vi "Example Write File - Allocate String.vi"(8 "buffer":string, 9 "session id":i32, 10 "error in":errorcluster, 11 "reference in":refnum<k24>) -> (1 "string id":i32, 2 "error out":errorcluster, 3 "reference out":refnum<k24>)   [LabVIEW 2010]
uses:
  C:/tf/play/labview/Tinkerforge.dll
  Tinkerforge.dll
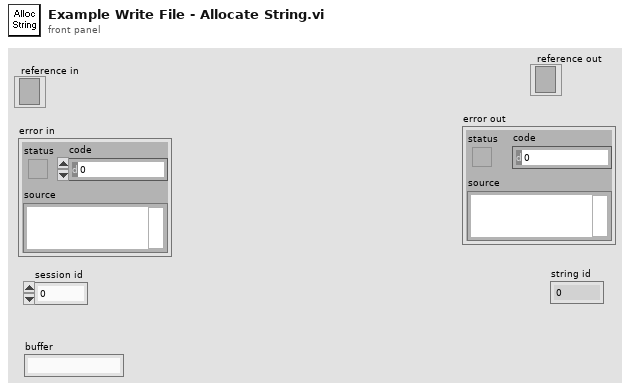
[diagram p1: front panel]
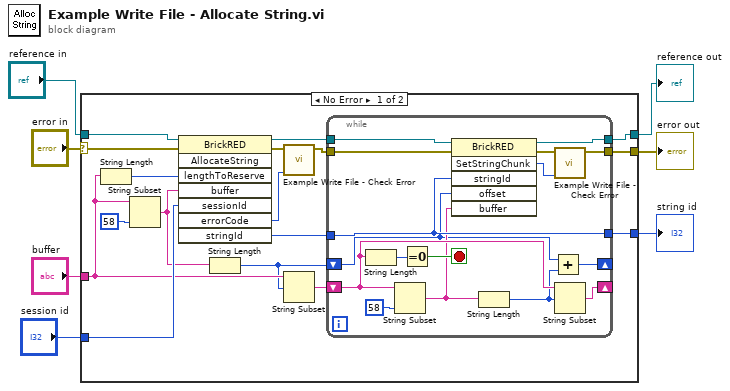
[diagram p0: block diagram]
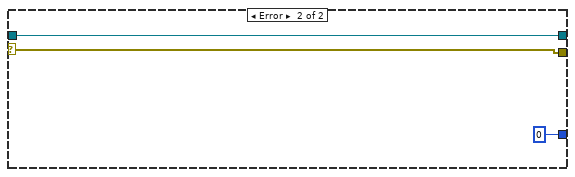
[diagram p2: hidden frame]
diagram:
  n1 = case shown="No Error" "error in" {
    selector: "error in" -> [w24 w43]
    tunnel: [w18 w43] -> w6
    tunnel: [w19 w42] -> w5
    tunnel: "reference in" -> [w23 w42]
    tunnel: "session id" -> [w22 _]
    tunnel: "buffer" -> [w15 _]
    tunnel: [w16 0 ("stringId")] -> w1
    frame No Error {
      n2 = String Length(string=w15) -> (length=w21:i32)
      n3 = String Subset(string=w15, length (rest)=58 ("length (rest)")) -> (substring=w12:string)  [unwired: 1 in]
      n4 = invoke class="BrickRED" method="AllocateString"(reference=w23, error in=w24, "lengthToReserve"=w21, "buffer"=w12, "sessionId"=w22) -> (reference out=w20:refnum<k24>, error out=w10:errorcluster, "errorCode"=w8:u8, "stringId"=w17:i32)  [unwired: 3 in, 4 out]
      n5 = String Length(string=w12) -> (length=w11:i32)
      n6 = call "Example Write File - Check Error.vi"("error code"=w8, "error in"=w10) -> ("error out"=w9:errorcluster)  [unwired: 9 in]
      n7 = String Subset(string=w15, offset (0)=w11) -> (substring=w13:string)  [unwired: 1 in]
      n8 = while {
        tunnel: w9 -> [w40]
        tunnel: [w26] -> w18
        tunnel: w20 -> [w39]
        tunnel: [w38] -> w19
        tunnel: w17 -> [w37]
        tunnel: [w37] -> w16
        shift-right: [w33] -> _
        shift-left: w13 -> [w32]
        shift-right: [w28] -> _
        shift-left: w11 -> [w30]
        stop <- w35 stop-if-true
        n9 = String Length(string=w32) -> (length=w36:i32)
        n10 = String Subset(string=w32, length (rest)=58) -> (substring=w31:string)  [unwired: 1 in]
        n11 = Equal To 0?(x=w36) -> (x = 0?=w35:bool)
        n12 = invoke class="BrickRED" method="SetStringChunk"(reference=w39, error in=w40, "stringId"=w37, "offset"=w30, "buffer"=w31) -> (reference out=w38:refnum<k24>, error out=w27:errorcluster, "SetStringChunk"=w25:u8)  [unwired: 1 in, 3 out]
        n13 = String Length(string=w31) -> (length=w29:i32)
        n14 = Add(x=w30, y=w29) -> (x+y=w28:i32)
        n15 = call "Example Write File - Check Error.vi"("error code"=w25, "error in"=w27) -> ("error out"=w26:errorcluster)  [unwired: 9 in]
        n16 = String Subset(string=w32, offset (0)=w29) -> (substring=w33:string)  [unwired: 1 in]
      }
    }
    frame Error {
    }
  }
  "error out" <- w6
  "reference out" <- w5
  "string id" <- w1
